vi "Configuration UI.vi"(11 "CSV Settings In":T1) -> (3 "CSV Settings Out":T1)   [LabVIEW 2022 SP3, in "CSV Export.lvlib" / "CSV Export.lvclass"]
uses:
  CSV Export.lvclass
  Controls/CSV Export Settings.ctl
panel:
  in  "Log Properties":bool caption="Log Channel Properties"
  in  "Log Units":bool caption="Log Channel Unit"
  in  "Use Relative Time":bool
  in  "Cancel":bool
  in  "OK":bool
  in  "Digits of Precision":u32=3 max=9
  in  "Log Stats":bool caption="Log Channel Statistics"
  in  "Resample":bool
  in  "Resample Rate (Hz)":dbl=100.0 min=0.0001 max=10000.0
  in  "Time Format":string
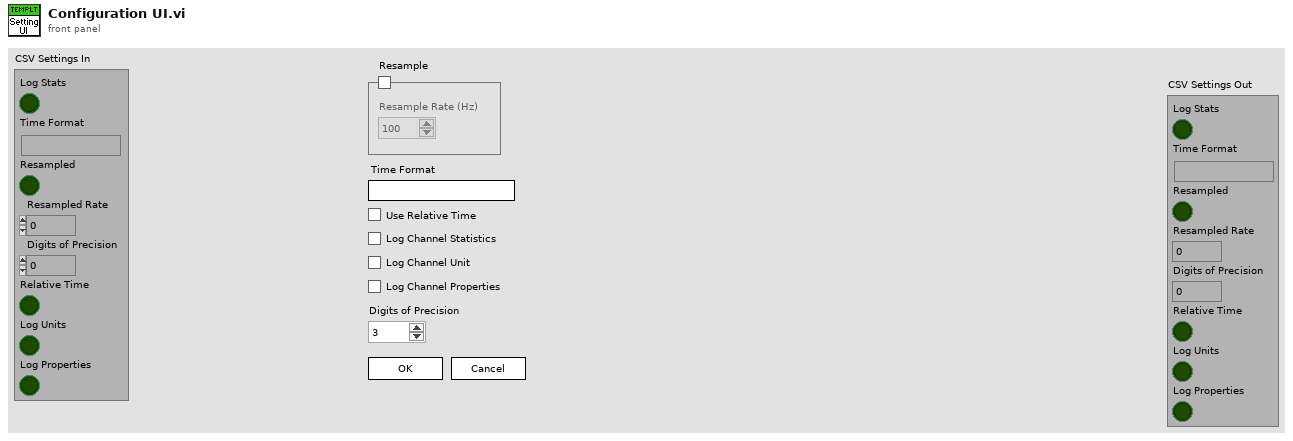
[diagram p1: front panel]
types:
  T1 = typedef "CSV Export.lvlib/CSV Export.lvclass/CSV Export Settings.ctl" = cluster{"Log Stats":bool, "Time Format":string, "Resampled":bool, "Resampled Rate":dbl, "Digits of Precision":u32, "Relative Time":bool, "Log Units":bool, "Log Properties":bool}
  T2 = enum32{"Invalid", "Standard", "Closed", "Hidden", "Minimized", "Maximized"}
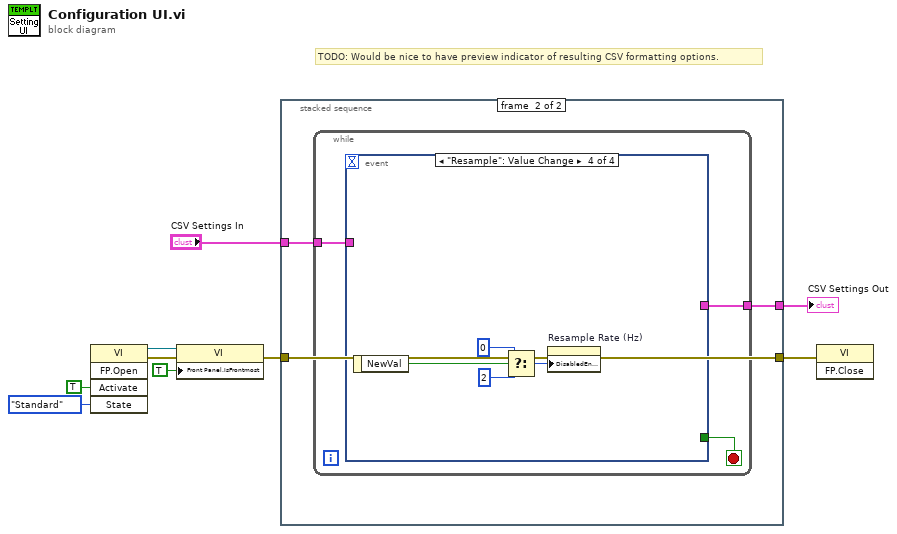
[diagram p0: block diagram]
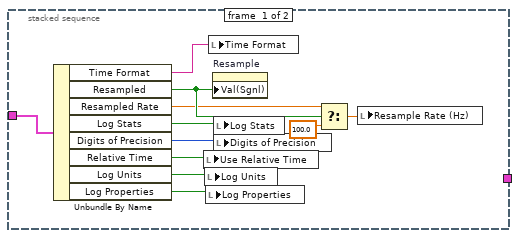
[diagram p2: hidden frame]
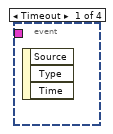
[diagram p3: hidden frame]
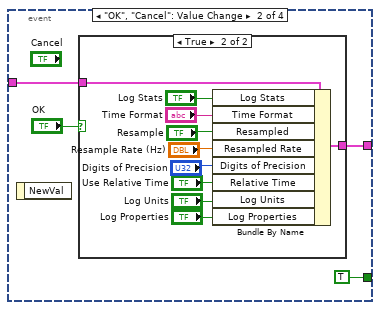
[diagram p4: hidden frame]
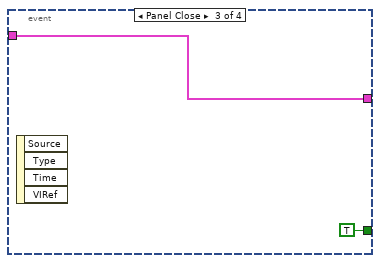
[diagram p6: hidden frame]
diagram:
  # "TODO: Would be nice to have preview indicator of resulting CSV formatting options."
  n1 = invoke class="VI" method="FP.Open"("Activate"=TRUE ("Activate?"), "State"=T2."Standard") -> (reference out=w3:refnum<vi>, error out=w2:errorcluster)  [unwired: 3 in, 3 out]
  n2 = property class="VI"(reference=w3, error in=w2, "Front Panel.IsFrontmost"=TRUE ("Front Panel Window:Is Frontmost")) -> (error out=w1:errorcluster)  [unwired: 1 out]
  n3 = stacked-sequence {
    tunnel: "CSV Settings In" -> [w19 w23]
    tunnel: [_ w22] -> w8
    tunnel: w1 -> [_ w21]
    tunnel: [_ w21] -> w5
    frame #0 {
      n4 = Unbundle By Name(w19) -> ("Time Format"=w20:string, "Resampled"=w15:bool, "Resampled Rate"=w14:dbl, "Log Stats"=w18:bool, "Digits of Precision"=w17:u32, "Relative Time"=w16:bool, "Log Units"=w11:bool, "Log Properties"=w10:bool)
      n5 = local write "Use Relative Time"(w16) -> ()
      n6 = local write "Log Units"(w11) -> ()
      n7 = local write "Log Properties"(w10) -> ()
      n8 = local write "Time Format"(w20) -> ()
      n9 = property on="Resample" class="Bool (strict)"("Val(Sgnl)"=w15) -> ()  [unwired: 2 in, 2 out]
      n10 = local write "Log Stats"(w18) -> ()
      n11 = local write "Digits of Precision"(w17) -> ()
      n12 = Select(t=w14, s=w15, f=100.0) -> (s? t:f=w13:dbl)
      n13 = local write "Resample Rate (Hz)"(w13) -> ()
    }
    frame #1 {
      n14 = while {
        tunnel: w23 -> [w26]
        tunnel: [w24] -> w22
        stop <- w25 stop-if-true
        n15 = event shown="[3] \"Resample\": Value Change" {
          selector: _ -> [_ _ _ _]
          dyn-events: _ -> [_ _ _ _]
          timeout: _ -> [_ _ _ _]
          tunnel: w26 -> [_ w30 w43 _]
          tunnel: [_ TRUE TRUE _] -> w25
          tunnel: [_ w27 w43 _] -> w24
          event Timeout {
            n16 = event-data() -> ()  [unwired: 1 in, 3 out]
          }
          event "OK", "Cancel": Value Change {
            n17 = event-data() -> ()  [unwired: 1 in, 1 out]
            n18 = case shown="True" "OK" {
              tunnel: w30 -> [w31 w41]
              tunnel: [w31 w40] -> w27
              frame False {
              }
              frame True {
                n19 = Bundle By Name(cluster=w41, "Log Stats"="Log Stats", "Time Format"="Time Format", "Resampled"="Resample", "Resampled Rate"="Resample Rate (Hz)", "Digits of Precision"="Digits of Precision", "Relative Time"="Use Relative Time", "Log Units"="Log Units", "Log Properties"="Log Properties") -> (w40:T1)
              }
            }
          }
          event Panel Close {
            n20 = event-data() -> ()  [unwired: 1 in, 4 out]
          }
          event "Resample": Value Change {
            n21 = event-data() -> ("NewVal"=w46:bool)  [unwired: 1 in]
            n22 = Select(t=0, s=w46, f=2) -> (s? t:f=w44:i32)
            n23 = property on="Resample Rate (Hz)" class="DigNum (strict)"("DisabledEnum"=w44) -> ()  [unwired: 2 in, 2 out]
          }
        }
      }
    }
  }
  "CSV Settings Out" <- w8
  n24 = invoke class="VI" method="FP.Close"(error in=w5) -> ()  [unwired: 2 in, 3 out]
